vi "User Interface Event Handler.vi"() -> ()   [LabVIEW 2020]
uses:
  <vilib>/DAQmx/miscellaneous.llb/DAQmx Fill In Error Info.vi
  <vilib>/DAQmx/write.llb/DAQmx Write (Analog DBL 1Chan 1Samp).vi
  <vilib>/DAQmx/read.llb/DAQmx Read (Analog 2D DBL NChan NSamp).vi
  <vilib>/DAQmx/create/channels.llb/DAQmx Create Channel (AO-Voltage-Basic).vi
  <vilib>/Utility/file.llb/Write Delimited Spreadsheet (DBL).vi
  <vilib>/DAQmx/create/channels.llb/DAQmx Create Channel (AI-Voltage-Basic).vi
  <vilib>/DAQmx/configure/timing.llb/DAQmx Timing (Sample Clock).vi
panel:
  in  "Generate Stimulus":bool
  in  "AO Voltage Channel":tag="PCI-6221/ao0"
  in  "Analyze":bool
  in  "Save Data":bool
  in  "Clear":bool
  in  "Exit":bool
  in  "Acquire":bool
  in  "Samples per channel":i32=100
  in  "Sample Rate":dbl=1000.0
  in  "AI Voltage Channel":tag="PCI-6221/ai0, PCI-6221/ai3"
  out "Graph":dbl[][](graph)
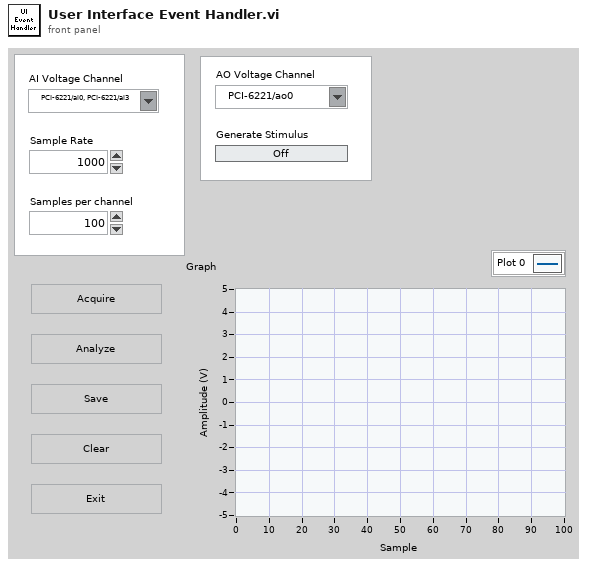
[diagram p1: front panel]
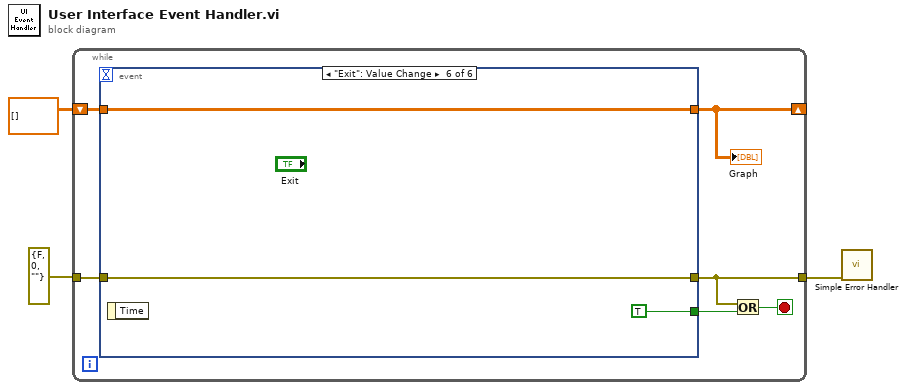
[diagram p0: block diagram]
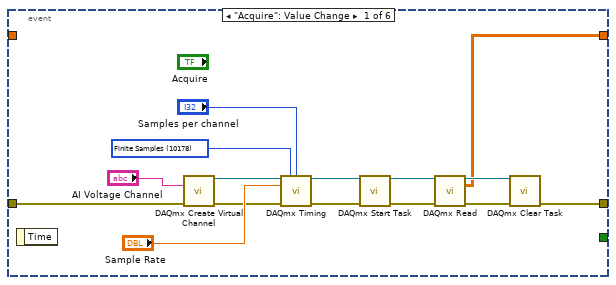
[diagram p2: hidden frame]
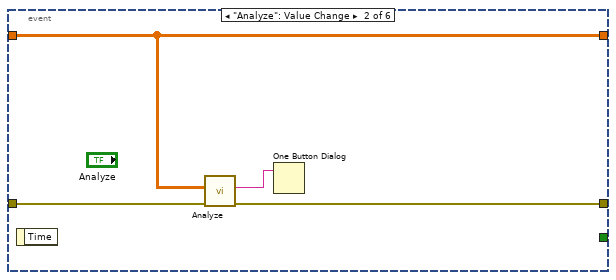
[diagram p3: hidden frame]
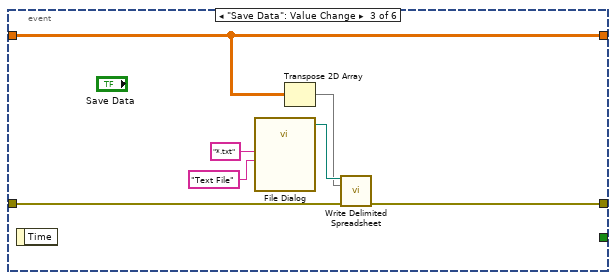
[diagram p4: hidden frame]
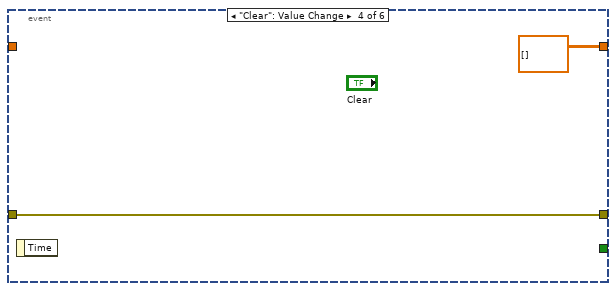
[diagram p5: hidden frame]
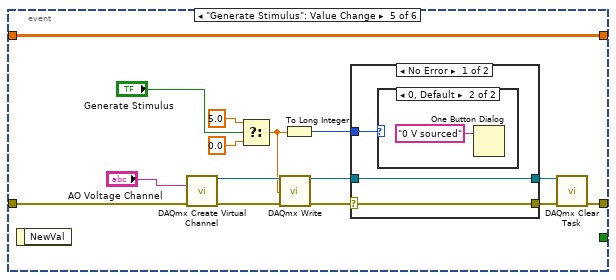
[diagram p6: hidden frame]
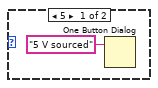
[diagram p7: hidden frame]
diagram:
  n1 = while {
    shift-right: [w5] -> _
    shift-left: dbl[][] [] -> [w6]
    tunnel: errorcluster {"status"=FALSE, "code"=0, "source"=""} ("error constant") -> [w8]
    tunnel: [w7] -> w3
    stop <- w9 stop-if-true
    n2 = event shown="[5] \"Exit\": Value Change" {
      selector: _ -> [_ _ _ _ _ _]
      dyn-events: _ -> [_ _ _ _ _ _]
      timeout: _ -> [_ _ _ _ _ _]
      tunnel: w8 -> [w11 w28 w29 w37 w38 w62]
      tunnel: [w10 w27 w30 w37 w40 w62] -> w7
      tunnel: w6 -> [_ w25 w31 _ w39 w60]
      tunnel: [w12 w25 w31 dbl[][] [] w39 w60] -> w5
      tunnel: [_ _ _ _ _ TRUE] -> w4
      event "Acquire": Value Change {
        w13 = 10178 items=["Finite Samples"=10178, "Continuous Samples"=10123, "Hardware Timed Single Point"=12522] ("sample mode")
        n3 = event-data() -> ()  [unwired: 1 in, 1 out]
        n4 = call-poly <vilib>:"DAQmx Create Virtual Channel.vi"("physical channels"="AI Voltage Channel", "error in"=w11) -> ("task out"=w14:refnum<k21>, "error out"=w15:errorcluster)  [unwired: 12 in]
        n5 = call-poly <vilib>:"DAQmx Timing.vi"("task/channels in"=w14, "sample mode"=w13, "samples per channel"="Samples per channel", "rate"="Sample Rate", "error in"=w15) -> ("task out"=w16:refnum<k21>, "error out"=w17:errorcluster)  [unwired: 9 in]
        n6 = call <vilib>:"DAQmx Start Task.vi"("task/channels in"=w16, "error in"=w17) -> ("task out"=w18:refnum<k21>, "error out"=w19:errorcluster)  [unwired: 12 in]
        n7 = call-poly <vilib>:"DAQmx Read.vi"("task/channels in"=w18, "error in"=w19) -> ("task out"=w20:refnum<k21>, "data"=w12:dbl[][], "error out"=w21:errorcluster)  [unwired: 11 in]
        n8 = call <vilib>:"DAQmx Clear Task.vi"("task in"=w20, "error in"=w21) -> ("error out"=w10:errorcluster)  [unwired: 13 in]
      }
      event "Analyze": Value Change {
        n9 = event-data() -> ()  [unwired: 1 in, 1 out]
        n10 = call "Analyze.vi"("error in"=w28, "n-channel data (2D DBL)"=w25) -> ("error out"=w27:errorcluster, "message"=w26:string)  [unwired: 6 in]
        n11 = One Button Dialog(message=w26) -> ()  [unwired: 1 in, 1 out]
      }
      event "Save Data": Value Change {
        n12 = event-data() -> ()  [unwired: 1 in, 1 out]
        n13 = call "File Dialog"("pattern (all files)"="*.txt", "pattern label"="Text File") -> ("selected path"=w35:path)  [unwired: 10 in, 3 out]
        n14 = Transpose 2D Array(2D array=w31) -> (transposed array=w34:dbl[][])
        n15 = call-poly <vilib>:"Write Delimited Spreadsheet.vi"("file path (dialog if empty)"=w35, "2D data"=w34, "error in (no error)"=w29) -> ("error out"=w30:errorcluster)  [unwired: 11 in, 1 out]
      }
      event "Clear": Value Change {
        n16 = event-data() -> ()  [unwired: 1 in, 1 out]
      }
      event "Generate Stimulus": Value Change {
        n17 = event-data() -> ()  [unwired: 1 in, 1 out]
        n18 = call-poly <vilib>:"DAQmx Create Virtual Channel.vi"("physical channels"="AO Voltage Channel", "error in"=w38) -> ("task out"=w51:refnum<k21>, "error out"=w52:errorcluster)  [unwired: 12 in]
        n19 = Select(t=5.0, s="Generate Stimulus", f=0.0) -> (s? t:f=w47:dbl)
        n20 = call-poly <vilib>:"DAQmx Write.vi"("task/channels in"=w51, "data"=w47, "error in"=w52) -> ("task out"=w43:refnum<k21>, "error out"=w44:errorcluster)  [unwired: 10 in, 1 out]
        n21 = To Long Integer(number=w47) -> (32bit integer=w48:i32)
        n22 = case shown="No Error" w44 {
          selector: w44 -> [w53 w59]
          tunnel: w48 -> [w55 _]
          tunnel: w43 -> [w54 w58]
          tunnel: [w54 w58] -> w42
          tunnel: [w53 w59] -> w41
          frame No Error {
            n23 = case shown="0, Default" w55 {
              frame 5 {
                n24 = One Button Dialog(message="5 V sourced") -> ()  [unwired: 1 in, 1 out]
              }
              frame 0, Default {
                n25 = One Button Dialog(message="0 V sourced") -> ()  [unwired: 1 in, 1 out]
              }
            }
          }
          frame Error {
          }
        }
        n26 = call <vilib>:"DAQmx Clear Task.vi"("task in"=w42, "error in"=w41) -> ("error out"=w40:errorcluster)  [unwired: 13 in]
      }
      event "Exit": Value Change {
        n27 = event-data() -> ()  [unwired: 1 in, 1 out]
      }
    }
    "Graph" <- w5
    n28 = Or(x=w7, y=w4) -> (x .or. y?=w9:bool)
  }
  n29 = call <vilib>:"Simple Error Handler.vi"("error in (no error)"=w3) -> ()  [unwired: 4 in, 5 out]
